vi "Read CSM States By CSM-VI.vi"(6 "Config Path":path, 8 "Error In":errorcluster caption="Error in (no error)", 11 "CSM VI":string) -> (0 "Error Out":errorcluster, 3 "Array":string[](array[string]))   [LabVIEW 2017, in "CSM-Helper API with lvcsm Support.lvlib"]
uses:
  CSM-Helper API with lvcsm Support.lvlib
  lvcsmFile/lvcsm File Support.lvlib
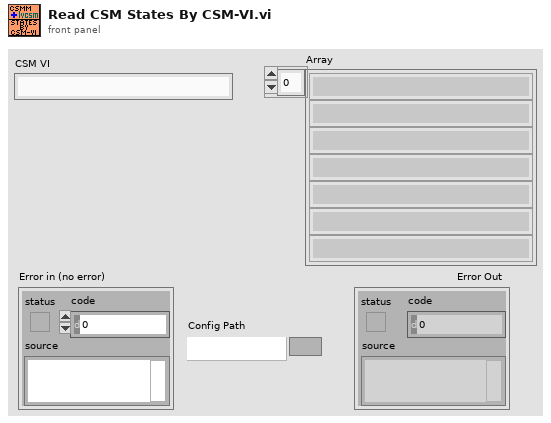
[diagram p1: front panel]
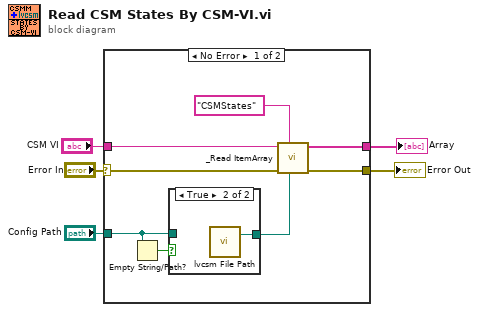
[diagram p0: block diagram]
diagram:
  n1 = case shown="No Error" "Error In" {
    selector: "Error In" -> [w11 w16]
    tunnel: [w10 w16] -> w4
    tunnel: "Config Path" -> [w13 _]
    tunnel: [w9 _] -> w2
    tunnel: "CSM VI" -> [w7 _]
    frame No Error {
      n2 = Empty String/Path?(string/path=w13) -> (empty?=w12:bool)
      n3 = case shown="True" w12 {
        tunnel: [w14 w15] -> w6
        tunnel: w13 -> [w14 _]
        frame False {
        }
        frame True {
          n4 = call "lvcsm File Path.vi"() -> ("Appended Path"=w15:path)  [unwired: 3 in]
        }
      }
      n5 = call "_Read ItemArray.vi"("Config Path"=w6, "Section Prefix"="CSMStates" ("Section"), "Error In"=w11, "Section"=w7) -> ("Error Out"=w10:errorcluster, "Array"=w9:string[])  [unwired: 6 in]
    }
    frame Error {
    }
  }
  "Error Out" <- w4
  "Array" <- w2
